vi "readFromXML.vi"(8 "error in (no error)":errorcluster, 10 "XML in":string, 11 "instrumentSelect in":refnum<class "InstrumentSelect.lvclass">) -> (0 "error out":errorcluster, 3 "instrumentSelect out":refnum<class "InstrumentSelect.lvclass">)   [LabVIEW 2014, in "TCSDataDefinitions.lvlib" / "TCSCommand.lvlib" / "InstrumentSelect.lvclass"]
uses:
  InstrumentSelect.lvclass
  InstrumentSelect.lvclass/InstrumentSelect.ctl
  TCSTcsCommand/TCSTcsCommand.lvclass
  <userlib>/Common/XML/XMLParser/XMLParser.lvclass
panel:
  out "instrumentName":string
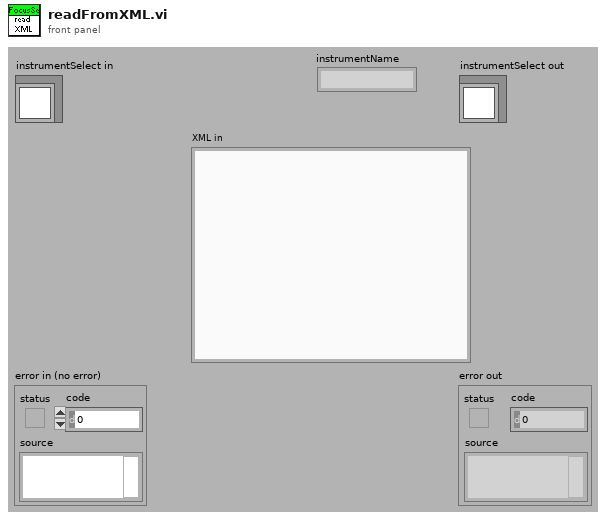
[diagram p1: front panel]
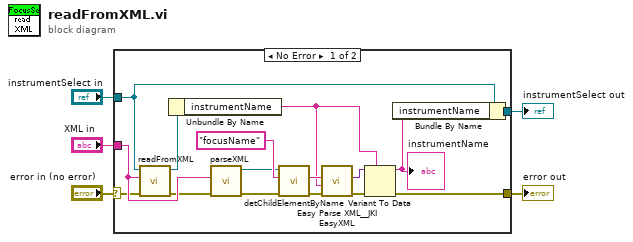
[diagram p0: block diagram]
diagram:
  n1 = case shown="No Error" "error in (no error)" {
    selector: "error in (no error)" -> [w8 w22]
    tunnel: [w12 w23] -> w3
    tunnel: "instrumentSelect in" -> [w11 w23]
    tunnel: "XML in" -> [w9 _]
    tunnel: [w13 w22] -> w1
    frame No Error {
      n2 = call-parent "readFromXML.vi"("error in (no error)"=w8, "XMLin"=w9, "TCSTcsCommand in"=w11) -> ("error out"=w7:errorcluster, "TCSTcsCommand out"=w10:refnum<class "InstrumentSelect.lvclass">)  [unwired: 7 in]
      n3 = Unbundle By Name(w10) -> ("instrumentName"=w15:string)
      n4 = call <userlib>:"parseXML.vi"("error in (no error)"=w7, "XMLString in"=w9) -> ("error out"=w21:errorcluster, "Element out"=w6:refnum<class "XMLParser.lvclass">)  [unwired: 8 in]
      n5 = call <userlib>:"detChildElementByName.vi"("error in (no error)"=w21, "childName"="focusName" ("ChildName"), "Element in"=w6) -> ("error out"=w18:errorcluster, "childXML"=w19:string)  [unwired: 5 in, 2 out]
      n6 = call <vilib>:"Easy Parse XML__JKI EasyXML.vi"("error in (no error)"=w18, "LabVIEW Data (Type)"=w15, "XML String"=w19) -> ("error out"=w17:errorcluster, "LabVIEW Data"=w16:variant)  [unwired: 7 in]
      n7 = Variant To Data(error in=w17, type=w15, Variant=w16) -> (data=w14:string, error out=w13:errorcluster)
      "instrumentName" <- w14
      n8 = Bundle By Name(cluster=w11, "instrumentName"=w14) -> (w12:refnum<class "InstrumentSelect.lvclass">)
    }
    frame Error {
    }
  }
  "error out" <- w1
  "instrumentSelect out" <- w3
